vi "Write connection ID.vi"(10 "connection ID":i32, 11 "Task in":refnum<class "Channel.lvclass">) -> (3 "Task out":refnum<class "Channel.lvclass">)   [LabVIEW 2009, in "MicroDAQ.lvlib" / "Channel.lvclass"]
uses:
  <instrlib>/MicroDAQ/Channel/Channel.lvclass
  <instrlib>/MicroDAQ/Channel/Channel.lvclass/Channel.ctl
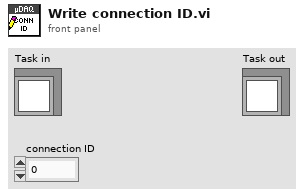
[diagram p1: front panel]
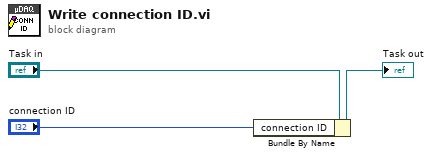
[diagram p0: block diagram]
diagram:
  n1 = Bundle By Name(cluster="Task in", "connection ID"="connection ID") -> (→"Task out":refnum<class "Channel.lvclass">)
